vi "Do_Every_minute.vi"(1 "Ch Names":string[](array[string]), 2 "Values":dbl[](array[numeric]) format="%.2f") -> ()   [LabVIEW 2010]
uses:
  Do_Every_5mins.ctl
  Anemometry/Anemometry Sub Vis/Controls/In_Range.ctl
  ADAM Client/Sub VIs/ADAM Controls/Traverse_Level_State.ctl
  ADAM Client/Sub VIs/ADAM Controls/Valco_valve_ph.ctl
  ADAM_Global.vi
panel:
  out "Case":T1
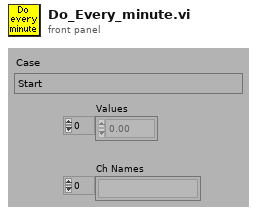
[diagram p1: front panel]
types:
  T1 = typedef "Do_Every_5mins.ctl" = enum16{"Start", "Update EnFlo Tunnel Speed Tweak", "Are EnFlo Tun Fan Bearings too Hot?", "Check EnFlo tweak factor?", "Are Inlet Screens Blocked?", "Tweak demanded chilled water temp", "Is Dew point meter Alive?", "Condensation Occurring", "Condensation Alert", "More checks", "Set FFID Valve to Measure", "End"}
  T2 = typedef "In_Range.ctl" = enum16{"%", "±", "% & ±"}
  T3 = typedef "Traverse_Level_State.ctl" = enum16{"Running", "Complete"}
  T4 = typedef "Client_State_Cluster.ctl" = cluster{"Client Name":string, "Traverse level State":T3, "People to Email":string[], "Next Contact Time":dbl}
  T5 = typedef "Valco_valve_ph.ctl" = u16
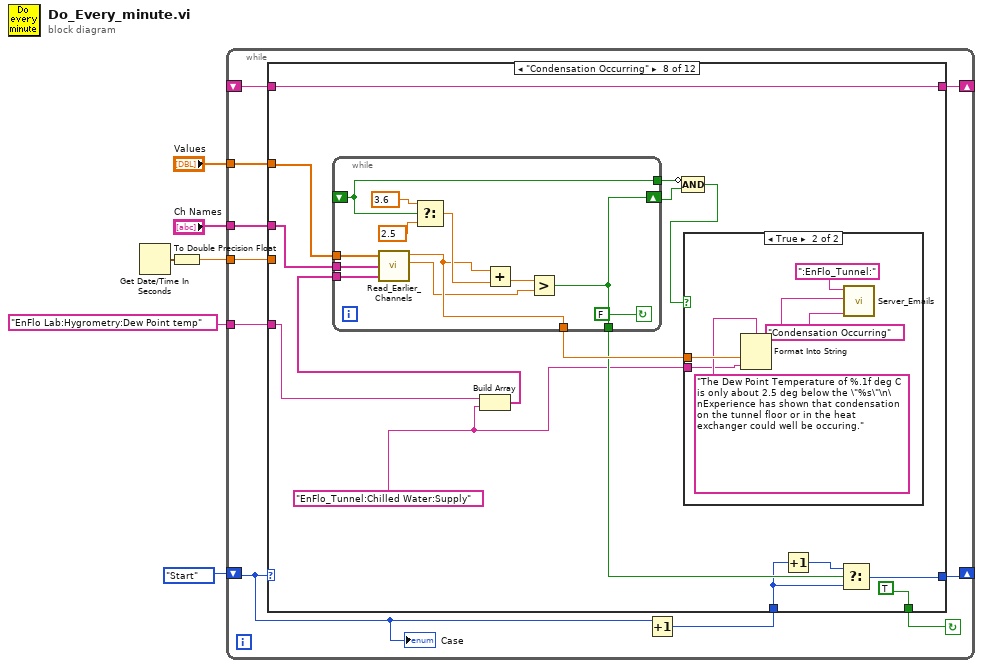
[diagram p0: block diagram]
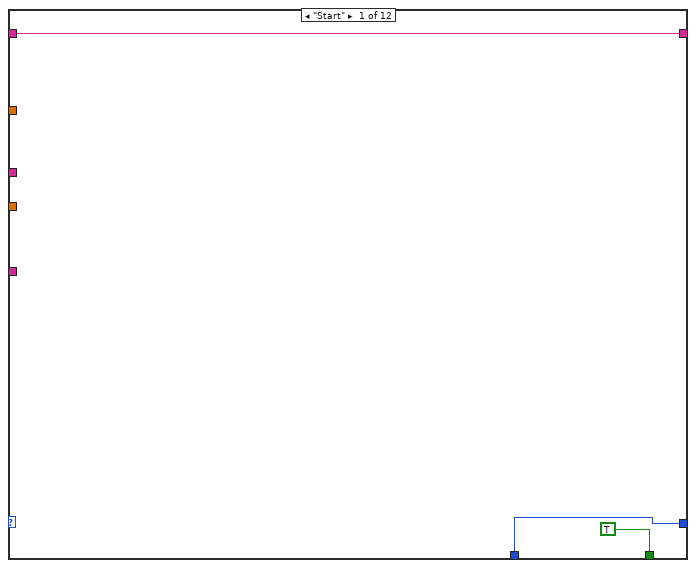
[diagram p2: hidden frame]
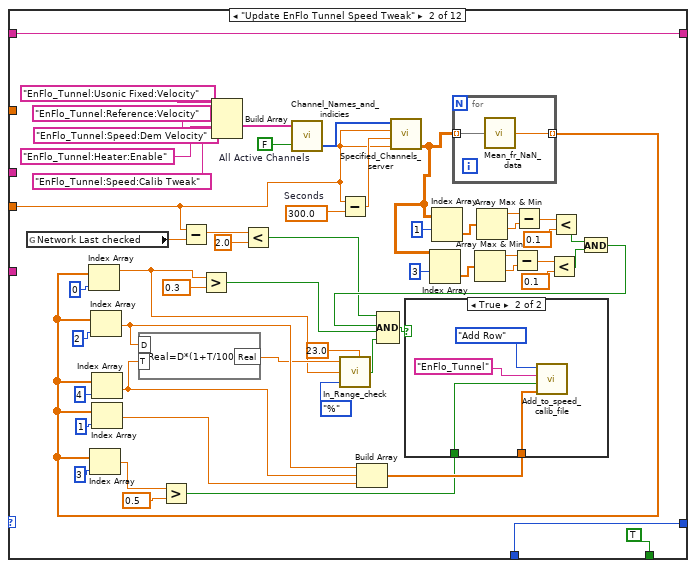
[diagram p3: hidden frame]
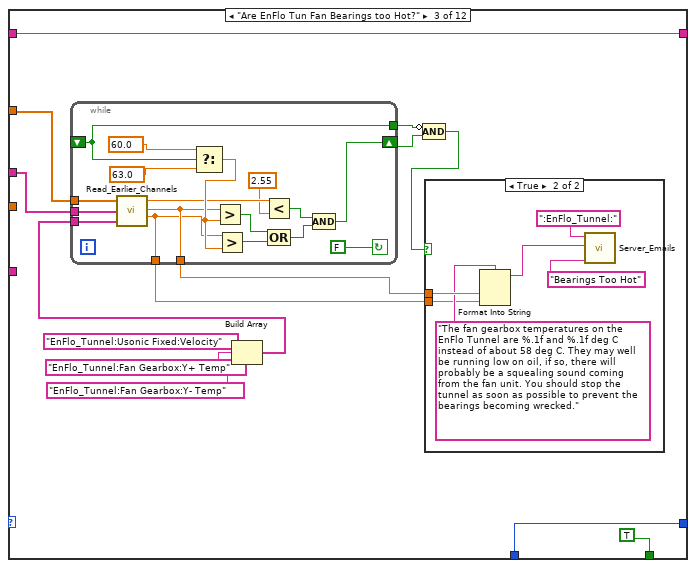
[diagram p5: hidden frame]
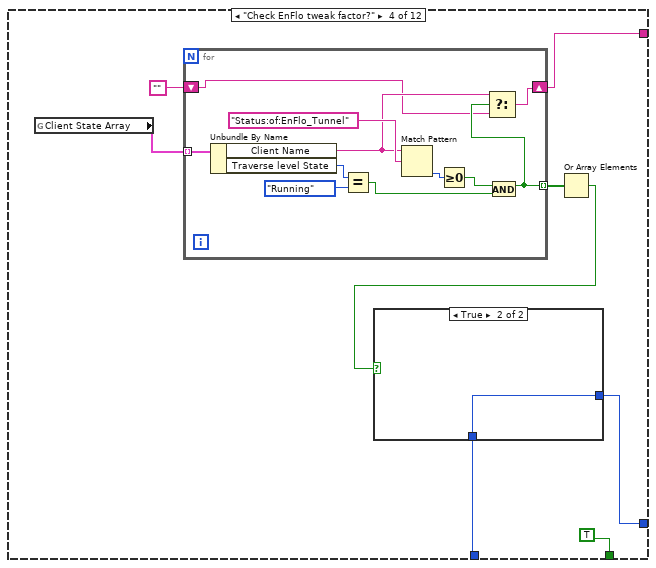
[diagram p7: hidden frame]
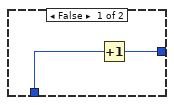
[diagram p8: hidden frame]
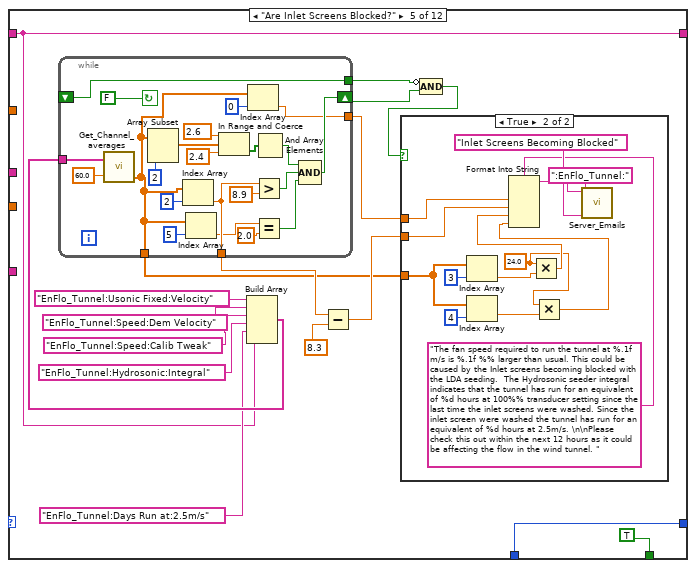
[diagram p9: hidden frame]
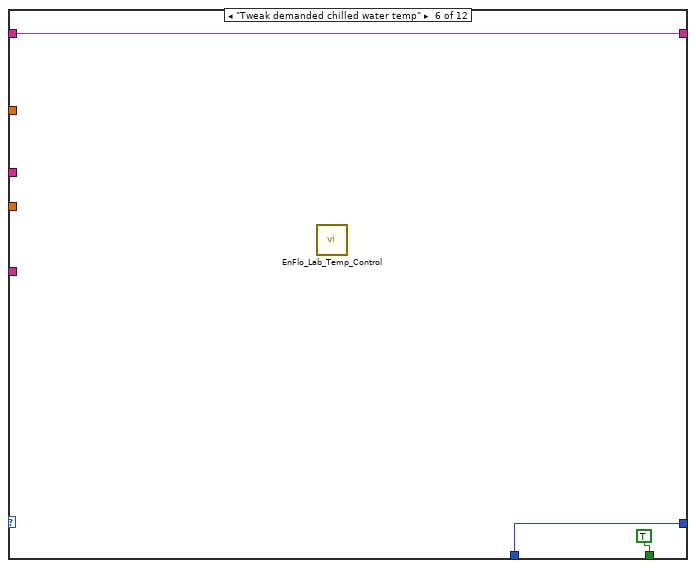
[diagram p11: hidden frame]
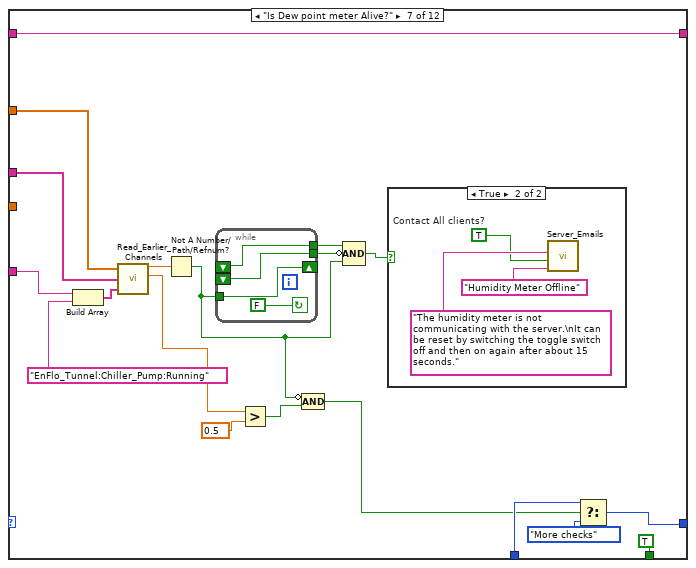
[diagram p12: hidden frame]
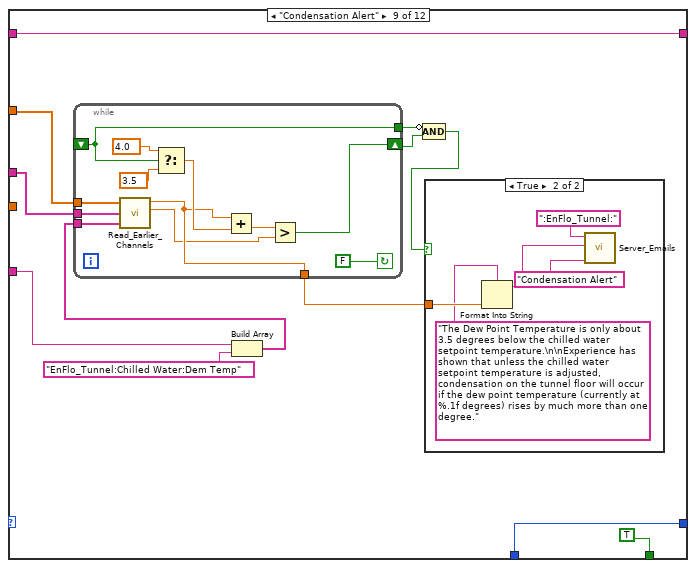
[diagram p15: hidden frame]
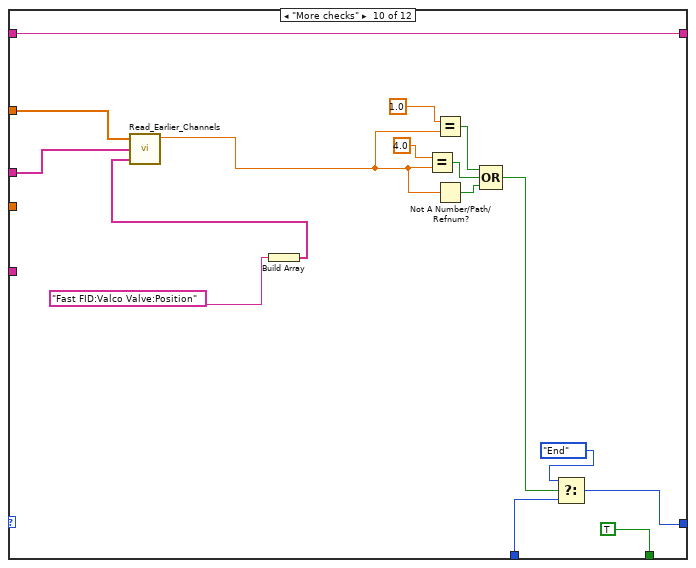
[diagram p17: hidden frame]
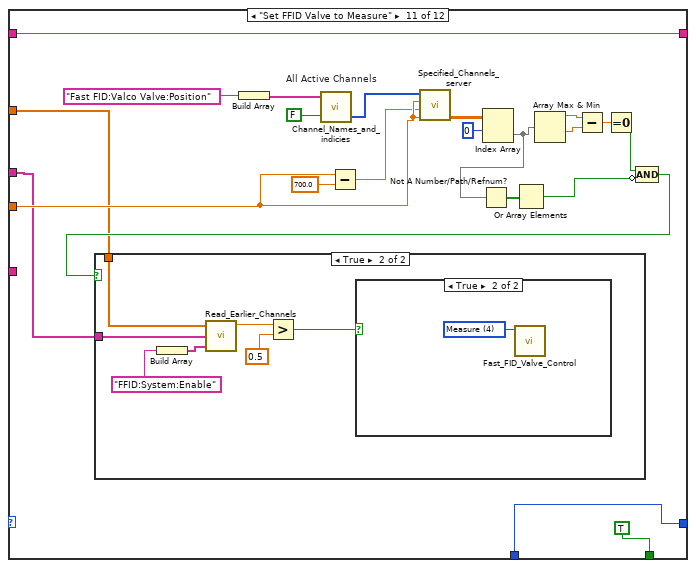
[diagram p18: hidden frame]
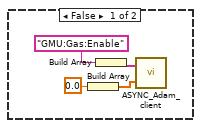
[diagram p20: hidden frame]
diagram:
  n1 = Get Date/Time In Seconds() -> (seconds since 1Jan1904=w2:timestamp)
  n2 = To Double Precision Float(number=w2) -> (double precision float=w1:dbl)
  n3 = while {
    tunnel: "EnFlo Lab:Hygrometry:Dew Point temp" -> [w10]
    tunnel: "Values" -> [w14]
    tunnel: "Ch Names" -> [w15]
    shift-left: Do_Every_5mins."Start" ("Case") -> [w11]
    shift-right: [w12] -> _
    tunnel: w1 -> [w9]
    shift-right: [w8] -> _
    shift-left: _ -> [w7]
    stop <- w16 continue-if-true
    n4 = Increment(x=w11) -> (x+1=w13:T1)
    n5 = case shown="\"Condensation Occurring\"" w11 {
      tunnel: [TRUE TRUE TRUE TRUE TRUE TRUE TRUE TRUE TRUE TRUE TRUE FALSE] -> w16
      tunnel: w15 -> [_ _ w91 _ _ _ w210 w234 w262 w297 w301 _]
      tunnel: w14 -> [_ _ w92 _ _ _ w211 w235 w263 w298 w300 _]
      tunnel: w13 -> [w17 w62 w82 w122 w149 w195 w202 w225 w265 w294 w320 w335]
      tunnel: [w17 w62 w82 w121 w149 w195 w214 w226 w265 w293 w320 w335] -> w12
      tunnel: w10 -> [_ _ _ _ _ _ w209 w228 w256 _ _ _]
      tunnel: w9 -> [_ w21 _ _ _ _ _ _ _ _ w318 _]
      tunnel: [w18 w25 w81 w118 w140 w193 w196 w223 w255 w296 w319 w336] -> w8
      tunnel: w7 -> [w18 w25 w81 _ w140 w193 w196 w223 w255 w296 w319 w336]
      frame "Start" {
      }
      frame "Update EnFlo Tunnel Speed Tweak" {
        w56 = 300.0  # Seconds
        w58 = FALSE  # All Active Channels
        n6 = global read "ADAM_Global.vi" "Network Last checked"() -> (w22:dbl)
        n7 = Subtract(x=w21, y=w22) -> (x-y=w23:dbl)
        n8 = Build Array("EnFlo_Tunnel:Usonic Fixed:Velocity", "EnFlo_Tunnel:Reference:Velocity", "EnFlo_Tunnel:Speed:Dem Velocity", "EnFlo_Tunnel:Heater:Enable", "EnFlo_Tunnel:Speed:Calib Tweak") -> (w55:string[])
        n9 = Less?(x=w23, y=2.0) -> (x < y?=w20:bool)
        n10 = call "Channel_Names_and_indicies.vi"("All Active Channels"=w58, "Desired Ch Names"=w55) -> ("Indicies"=w57:i32[])  [unwired: 1 out]
        n11 = Subtract(x=w21, y=w56) -> (x-y=w54:dbl)
        n12 = call "Specified_Channels_server.vi"("End time"=w21, "Start time"=w54, "Clients time"=w21, "Requested channels"=w57) -> ("Output array"=w36:dbl[][])  [unwired: 1 in, 4 out]
        n13 = Index Array(array=w36, index (row)=3 ("Index")) -> (element=w38:dbl[])  [unwired: 1 in]
        n14 = Index Array(array=w36, index (row)=1 ("Index")) -> (element=w52:dbl[])  [unwired: 1 in]
        n15 = for {
          tunnel: w36 -> [w76] mode=indexing
          tunnel: [w75] -> w45 mode=indexing
          n16 = call "Mean_fr_NaN_data.vi"("Data"=w76) -> ("Mean value"=w75:dbl)
        }
        n17 = Index Array(array=w45, index=0) -> (element=w29:dbl)
        n18 = Index Array(array=w45, index=3) -> (element=w65:dbl)
        n19 = Index Array(array=w45, index=2) -> (element=w31:dbl)
        n20 = Index Array(array=w45, index=4) -> (element=w32:dbl)
        n21 = Index Array(array=w45, index=1) -> (element=w43:dbl)
        n22 = formula code="Real=D*(1+T/100);"("D"=w31, "T"=w32) -> ("Real"=w30:dbl)
        n23 = Greater?(x=w65, y=0.5) -> (0:w44:bool)
        n24 = Greater?(x=w29, y=0.3) -> (0:w63:bool)
        n25 = call "In_Range_check.vi"("%"=23.0, "Mode"=In_Range."%", "Value"=w29, "Setpoint"=w30) -> ("In Range"=w26:bool)  [unwired: 1 in, 2 out]
        n26 = Build Array(w31, w32, w43) -> (w60:dbl[])
        n27 = Array Max & Min(array=w38) -> (max value=w39:dbl, min value=w40:dbl)  [unwired: 2 out]
        n28 = Array Max & Min(array=w52) -> (max value=w51:dbl, min value=w50:dbl)  [unwired: 2 out]
        n29 = Subtract(x=w39, y=w40) -> (x-y=w41:dbl)
        n30 = Subtract(x=w51, y=w50) -> (x-y=w49:dbl)
        n31 = Less?(x=w41, y=0.1) -> (x < y?=w35:bool)
        n32 = Less?(x=w49, y=0.1) -> (x < y?=w34:bool)
        n33 = And(x=w34, y=w35) -> (x .and. y?=w33:bool)
        n34 = Compound Arithmetic op=AND(w20, w33, w63, w26) -> (w59:bool)
        n35 = case shown="True" w59 {
          tunnel: w60 -> [_ w79]
          tunnel: w44 -> [_ w78]
          frame False {
          }
          frame True {
            n36 = call "Add_to_speed_calib_file.vi"("New Row"=w79, "Tunnel Heated?"=w78, "Rig Name"="EnFlo_Tunnel" ("y"), "Mode"=enum16{"Add Row", "Get Error Value"}."Add Row") -> ()  [unwired: 2 in, 2 out]
          }
        }
      }
      frame "Are EnFlo Tun Fan Bearings too Hot?" {
        n37 = Build Array("EnFlo_Tunnel:Usonic Fixed:Velocity", "EnFlo_Tunnel:Fan Gearbox:Y+ Temp", "EnFlo_Tunnel:Fan Gearbox:Y- Temp") -> (w90:string[])
        n38 = while {
          tunnel: [w96] -> w83
          tunnel: [w97] -> w84
          tunnel: [w106] -> w89
          shift-left: _ -> [w106]
          shift-right: [w98] -> w88
          tunnel: w90 -> [w109]
          tunnel: w91 -> [w110]
          tunnel: w92 -> [w111]
          stop <- FALSE continue-if-true
          n39 = call "Read_Earlier_Channels.vi"("Present scan array"=w111, "Ch names"=w110, "Desired Channels"=w109) -> ("Index 0"=w104:dbl, "Index 1"=w97:dbl, "Index 2"=w96:dbl)  [unwired: 3 out]
          n40 = Select(t=60.0, s=w106, f=63.0) -> (s? t:f=w105:dbl)
          n41 = Greater?(x=w97, y=w105) -> (0:w102:bool)
          n42 = Greater?(x=w96, y=w105) -> (0:w101:bool)
          n43 = Less?(x=w104, y=2.55) -> (x < y?=w100:bool)
          n44 = Compound Arithmetic op=OR(w102, w101) -> (w99:bool)
          n45 = Compound Arithmetic op=AND(w100, w99) -> (w98:bool)
        }
        n46 = Compound Arithmetic op=AND(invert w89, w88) -> (w87:bool)
        n47 = case shown="True" w87 {
          tunnel: w84 -> [_ w115]
          tunnel: w83 -> [_ w112]
          frame False {
          }
          frame True {
            n48 = Format Into String(format string="The fan gearbox temperatures on the EnFlo Tunnel are %.1f and %.1f deg C instead of about 58 deg C. They may well be running low on oil, if so, there will probably be a squealing sound coming from the fan unit. You should stop the tunnel as soon as possible to prevent the bearings becoming wrecked." ("Format String"), w115, w112) -> (resulting string=w114:string)  [unwired: 2 in, 1 out]
            n49 = call "Server_Emails.vi"("Client Name Contains"=":EnFlo_Tunnel:", "Message"=w114, "Subject"="Bearings Too Hot" ("Error Type")) -> ()  [unwired: 2 in, 3 out]
          }
        }
      }
      frame "Check EnFlo tweak factor?" {
        n50 = global read "ADAM_Global.vi" "Client State Array"() -> (w124:T4[])
        n51 = for {
          tunnel: w124 -> [w139] mode=indexing
          tunnel: [w132] -> w123 mode=indexing
          shift-right: [w130] -> w118
          shift-left: "" -> [w129]
          n52 = Unbundle By Name(w139) -> ("Client Name"=w131:string, "Traverse level State"=w138:T3)
          n53 = Equal?(x=w138, y=Traverse_Level_State."Running" ("Traverse level State")) -> (x = y?=w136:bool)
          n54 = Match Pattern(string=w131, regular expression="Status:of:EnFlo_Tunnel" ("y")) -> (offset past match=w134:i32)  [unwired: 4 out]
          n55 = Greater Or Equal To 0?(x=w134) -> (x >= 0?=w133:bool)
          n56 = And(x=w133, y=w136) -> (x .and. y?=w132:bool)
          n57 = Select(t=w131, s=w132, f=w129) -> (s? t:f=w130:string)
        }
        n58 = Or Array Elements(Boolean array=w123) -> (logical OR=w120:bool)
        n59 = case shown="True" w120 {
          tunnel: w122 -> [w127 w128]
          tunnel: [w126 w128] -> w121
          frame False {
            n60 = Increment(x=w127) -> (x+1=w126:T1)
          }
          frame True {
          }
        }
      }
      frame "Are Inlet Screens Blocked?" {
        n61 = Build Array("EnFlo_Tunnel:Usonic Fixed:Velocity", "EnFlo_Tunnel:Speed:Dem Velocity", "EnFlo_Tunnel:Speed:Calib Tweak", "EnFlo_Tunnel:Hydrosonic:Integral", "EnFlo_Tunnel:Days Run at:2.5m/s", w140) -> (w154:string[])
        n62 = while {
          tunnel: [w178] -> w153
          shift-left: _ -> [w178]
          shift-right: [w165] -> w152
          tunnel: w154 -> [w173]
          tunnel: [w164] -> w146
          tunnel: [w162] -> w145
          tunnel: [w160] -> w141
          stop <- FALSE continue-if-true
          n63 = call "Get_Channel_averages.vi"("Desired Ch Names"=w173, "Averaging time (mins)"=60.0) -> ("number"=w160:dbl[])  [unwired: 1 in, 2 out]
          n64 = Array Subset(array=w160, length=2) -> (w172:dbl[])  [unwired: 1 in]
          n65 = Index Array(array=w160, index=2) -> (element=w164:dbl)
          n66 = Index Array(array=w160, index=5) -> (element=w159:dbl)
          n67 = In Range and Coerce(upper limit=2.6 ("y"), x=w172, lower limit=2.4) -> (In Range?=w170:bool[])  [unwired: 1 out]
          n68 = Index Array(array=w160, index=0) -> (element=w162:dbl)
          n69 = Greater?(x=w164, y=8.9) -> (0:w167:bool)
          n70 = Equal?(x=w159, y=2.0) -> (x = y?=w157:bool)
          n71 = And Array Elements(Boolean array=w170) -> (logical AND=w166:bool)
          n72 = Compound Arithmetic op=AND(w166, w167, w157) -> (w165:bool)
        }
        n73 = Subtract(x=w146, y=8.3) -> (x-y=w144:dbl)
        n74 = Compound Arithmetic op=AND(invert w153, w152) -> (w151:bool)
        n75 = case shown="True" w151 {
          tunnel: w145 -> [_ w189]
          tunnel: w144 -> [_ w188]
          tunnel: w141 -> [_ w183]
          frame False {
          }
          frame True {
            w181 = 24.0 ("x")
            n76 = Index Array(array=w183, index=3) -> (element=w186:dbl)
            n77 = Index Array(array=w183, index=4) -> (element=w180:dbl)
            n78 = Multiply(x=w181, y=w186) -> (x*y=w182:dbl)
            n79 = Multiply(x=w181, y=w180) -> (x*y=w179:dbl)
            n80 = Format Into String(format string="The fan speed required to run the tunnel at %.1f m/s is %.1f %% larger than usual. This could be caused by the Inlet screens becoming blocked with the LDA seeding.  The Hydrosonic seeder integral indicates that the tunnel has run for an equivalent of %d hours at 100%% transducer setting since the last time the inlet screens were washed. Since the inlet screen were washed the tunnel has run for an equivalent of %d hours at 2.5m/s. \n\nPlease check this out within the next 12 hours as it could be affecting the flow in the wind tunnel. " ("Format String"), w189, w188, w182, w179) -> (resulting string=w190:string)  [unwired: 2 in, 1 out]
            n81 = call "Server_Emails.vi"("Client Name Contains"=":EnFlo_Tunnel:", "Message"=w190, "Subject"="Inlet Screens Becoming Blocked" ("Error Type")) -> ()  [unwired: 2 in, 3 out]
          }
        }
      }
      frame "Tweak demanded chilled water temp" {
        n82 = call "EnFlo_Lab_Temp_Control.vi"() -> ()  [unwired: 1 out]
      }
      frame "Is Dew point meter Alive?" {
        n83 = Build Array(w209, "EnFlo_Tunnel:Chiller_Pump:Running") -> (w207:string[])
        n84 = call "Read_Earlier_Channels.vi"("Present scan array"=w211, "Ch names"=w210, "Desired Channels"=w207) -> ("Index 0"=w206:dbl, "Index 1"=w204:dbl)  [unwired: 4 out]
        n85 = Not A Number/Path/Refnum?(number/path/refnum=w206) -> (NaN/Path/Refnum?=w199:bool)
        n86 = while {
          tunnel: [w216] -> w197
          tunnel: [w217] -> w198
          shift-left: _ -> [w217]
          tunnel: w199 -> [w218]
          shift-left: _ -> [w216]
          shift-right: [w218] -> _
          stop <- FALSE continue-if-true
        }
        n87 = Greater?(x=w204, y=0.5) -> (0:w203:bool)
        n88 = Compound Arithmetic op=AND(invert w199, w203) -> (w200:bool)
        n89 = Compound Arithmetic op=AND(w197, invert w198, w199) -> (w212:bool)
        n90 = case shown="True" w212 {
          frame False {
          }
          frame True {
            w219 = TRUE  # Contact All clients?
            n91 = call "Server_Emails.vi"("Message"="The humidity meter is not communicating with the server.\nIt can be reset by switching the toggle switch off and then on again after about 15 seconds." ("Bundle Element"), "Contact All clients?"=w219, "Subject"="Humidity Meter Offline" ("Error Type")) -> ()  [unwired: 2 in, 3 out]
          }
        }
        n92 = Select(t=w202, s=w200, f=Do_Every_5mins."More checks" ("Case")) -> (s? t:f=w214:T1)
      }
      frame "Condensation Occurring" {
        w222 = "EnFlo_Tunnel:Chilled Water:Supply"
        n93 = Build Array(w228, w222) -> (w233:string[])
        n94 = while {
          tunnel: [w238] -> w227
          tunnel: [w240] -> w229
          tunnel: [w241] -> w232
          shift-left: _ -> [w241]
          shift-right: [w238] -> w231
          tunnel: w233 -> [w246]
          tunnel: w234 -> [w247]
          tunnel: w235 -> [w248]
          stop <- FALSE continue-if-true
          n95 = call "Read_Earlier_Channels.vi"("Present scan array"=w248, "Ch names"=w247, "Desired Channels"=w246) -> ("Index 0"=w240:dbl, "Index 1"=w239:dbl)  [unwired: 4 out]
          n96 = Select(t=3.6, s=w241, f=2.5) -> (s? t:f=w242:dbl)
          n97 = Add(x=w240, y=w242) -> (x+y=w245:dbl)
          n98 = Greater?(x=w245, y=w239) -> (0:w238:bool)
        }
        n99 = Compound Arithmetic op=AND(invert w232, w231) -> (w230:bool)
        n100 = case shown="True" w230 {
          tunnel: w229 -> [_ w252]
          tunnel: w222 -> [_ w249]
          frame False {
          }
          frame True {
            n101 = Format Into String(format string="The Dew Point Temperature of %.1f deg C is only about 2.5 deg below the \"%s\"\n\nExperience has shown that condensation on the tunnel floor or in the heat exchanger could well be occuring." ("Format String"), w252, w249) -> (resulting string=w251:string)  [unwired: 2 in, 1 out]
            n102 = call "Server_Emails.vi"("Client Name Contains"=":EnFlo_Tunnel:", "Message"=w251, "Subject"="Condensation Occurring" ("Error Type")) -> ()  [unwired: 2 in, 3 out]
          }
        }
        n103 = Increment(x=w225) -> (x+1=w224:T1)
        n104 = Select(t=w224, s=w227, f=w225) -> (s? t:f=w226:T1)
      }
      frame "Condensation Alert" {
        n105 = Build Array(w256, "EnFlo_Tunnel:Chilled Water:Dem Temp") -> (w261:string[])
        n106 = while {
          tunnel: [w269] -> w257
          tunnel: [w271] -> w260
          shift-left: _ -> [w271]
          shift-right: [w270] -> w259
          tunnel: w261 -> [w276]
          tunnel: w262 -> [w277]
          tunnel: w263 -> [w278]
          stop <- FALSE continue-if-true
          n107 = call "Read_Earlier_Channels.vi"("Present scan array"=w278, "Ch names"=w277, "Desired Channels"=w276) -> ("Index 0"=w269:dbl, "Index 1"=w268:dbl)  [unwired: 4 out]
          n108 = Select(t=4.0, s=w271, f=3.5) -> (s? t:f=w272:dbl)
          n109 = Add(x=w269, y=w272) -> (x+y=w275:dbl)
          n110 = Greater?(x=w275, y=w268) -> (0:w270:bool)
        }
        n111 = Compound Arithmetic op=AND(invert w260, w259) -> (w258:bool)
        n112 = case shown="True" w258 {
          tunnel: w257 -> [_ w281]
          frame False {
          }
          frame True {
            n113 = Format Into String(format string="The Dew Point Temperature is only about 3.5 degrees below the chilled water setpoint temperature.\n\nExperience has shown that unless the chilled water setpoint temperature is adjusted, condensation on the tunnel floor will occur if the dew point temperature (currently at %.1f degrees) rises by much more than one degree." ("Format String"), w281) -> (resulting string=w280:string)  [unwired: 2 in, 1 out]
            n114 = call "Server_Emails.vi"("Client Name Contains"=":EnFlo_Tunnel:", "Message"=w280, "Subject"="Condensation Alert" ("Error Type")) -> ()  [unwired: 2 in, 3 out]
          }
        }
      }
      frame "More checks" {
        n115 = Build Array("Fast FID:Valco Valve:Position") -> (w291:string[])
        n116 = call "Read_Earlier_Channels.vi"("Present scan array"=w298, "Ch names"=w297, "Desired Channels"=w291) -> ("Index 0"=w284:dbl)  [unwired: 5 out]
        n117 = Equal?(x=4.0, y=w284) -> (x = y?=w288:bool)
        n118 = Equal?(x=1.0, y=w284) -> (x = y?=w287:bool)
        n119 = Not A Number/Path/Refnum?(number/path/refnum=w284) -> (NaN/Path/Refnum?=w289:bool)
        n120 = Compound Arithmetic op=OR(w287, w288, w289) -> (w286:bool)
        n121 = Select(t=Do_Every_5mins."End" ("Case"), s=w286, f=w294) -> (s? t:f=w293:T1)
      }
      frame "Set FFID Valve to Measure" {
        w317 = FALSE  # All Active Channels
        n122 = Build Array("Fast FID:Valco Valve:Position") -> (w315:string[])
        n123 = call "Channel_Names_and_indicies.vi"("All Active Channels"=w317, "Desired Ch Names"=w315) -> ("Indicies"=w316:i32[])  [unwired: 1 out]
        n124 = Subtract(x=w318, y=700.0) -> (x-y=w313:dbl)
        n125 = call "Specified_Channels_server.vi"("End time"=w318, "Start time"=w313, "Clients time"=w318, "Requested channels"=w316) -> ("Output array"=w310:dbl[][])  [unwired: 1 in, 4 out]
        n126 = Index Array(array=w310, index (row)=0 ("Index")) -> (element=w306:dbl[])  [unwired: 1 in]
        n127 = Not A Number/Path/Refnum?(number/path/refnum=w306) -> (NaN/Path/Refnum?=w305:bool[])
        n128 = Or Array Elements(Boolean array=w305) -> (logical OR=w303:bool)
        n129 = Array Max & Min(array=w306) -> (max value=w308:dbl, min value=w309:dbl)  [unwired: 2 out]
        n130 = Subtract(x=w308, y=w309) -> (x-y=w307:dbl)
        n131 = Equal To 0?(x=w307) -> (x = 0?=w304:bool)
        n132 = Compound Arithmetic op=AND(w304, invert w303) -> (w302:bool)
        n133 = case shown="True" w302 {
          tunnel: w301 -> [_ w328]
          tunnel: w300 -> [_ w327]
          frame False {
          }
          frame True {
            n134 = Build Array("FFID:System:Enable") -> (w325:string[])
            n135 = call "Read_Earlier_Channels.vi"("Present scan array"=w327, "Ch names"=w328, "Desired Channels"=w325) -> ("Index 0"=w324:dbl)  [unwired: 5 out]
            n136 = Greater?(x=w324, y=0.5) -> (0:w322:bool)
            n137 = case shown="True" w322 {
              frame False {
                n138 = Build Array(0.0) -> (w330:dbl[])
                n139 = Build Array("GMU:Gas:Enable") -> (w332:string[])
                n140 = call "ASYNC_Adam_client.vi"("Values"=w330, "Channel Names"=w332) -> ()  [unwired: 2 out]
              }
              frame True {
                w333 = T5 4 items=["", "Zero Air", "Calib 1", "Calib 2", "Measure"] ("Requested Position")
                n141 = call "Fast_FID_Valve_Control.vi"("Requested Position"=w333) -> ()  [unwired: 7 out]
              }
            }
          }
        }
      }
      frame "End" {
      }
    }
    "Case" <- w11
  }
